vi "课堂.vi"() -> ()   [LabVIEW 2025]
panel:
  out "循环次数 3":i32
  in  "停止 2":bool
  out "x^2":dbl
  in  "数值 2":dbl
  in  "标尺.范围:最小值":dbl
  in  "标尺.范围:最大值":dbl=900.0
  in  "停止":bool
  in  "显示宽度":dbl=100.0
  in  "滑动杆":dbl(slide) scale=0.0..900.0
  out "波形图":dbl[](graph)
  in  "循环次数":i32=1000
  out "x+1 2":dbl
  out "x+1":dbl
  in  "milliseconds to wait":u32=1000
  out "数值":dbl
  out "循环次数":i32
  in  "下限":dbl=49.0
  in  "上限":dbl=51.0
  out "x/y":dbl
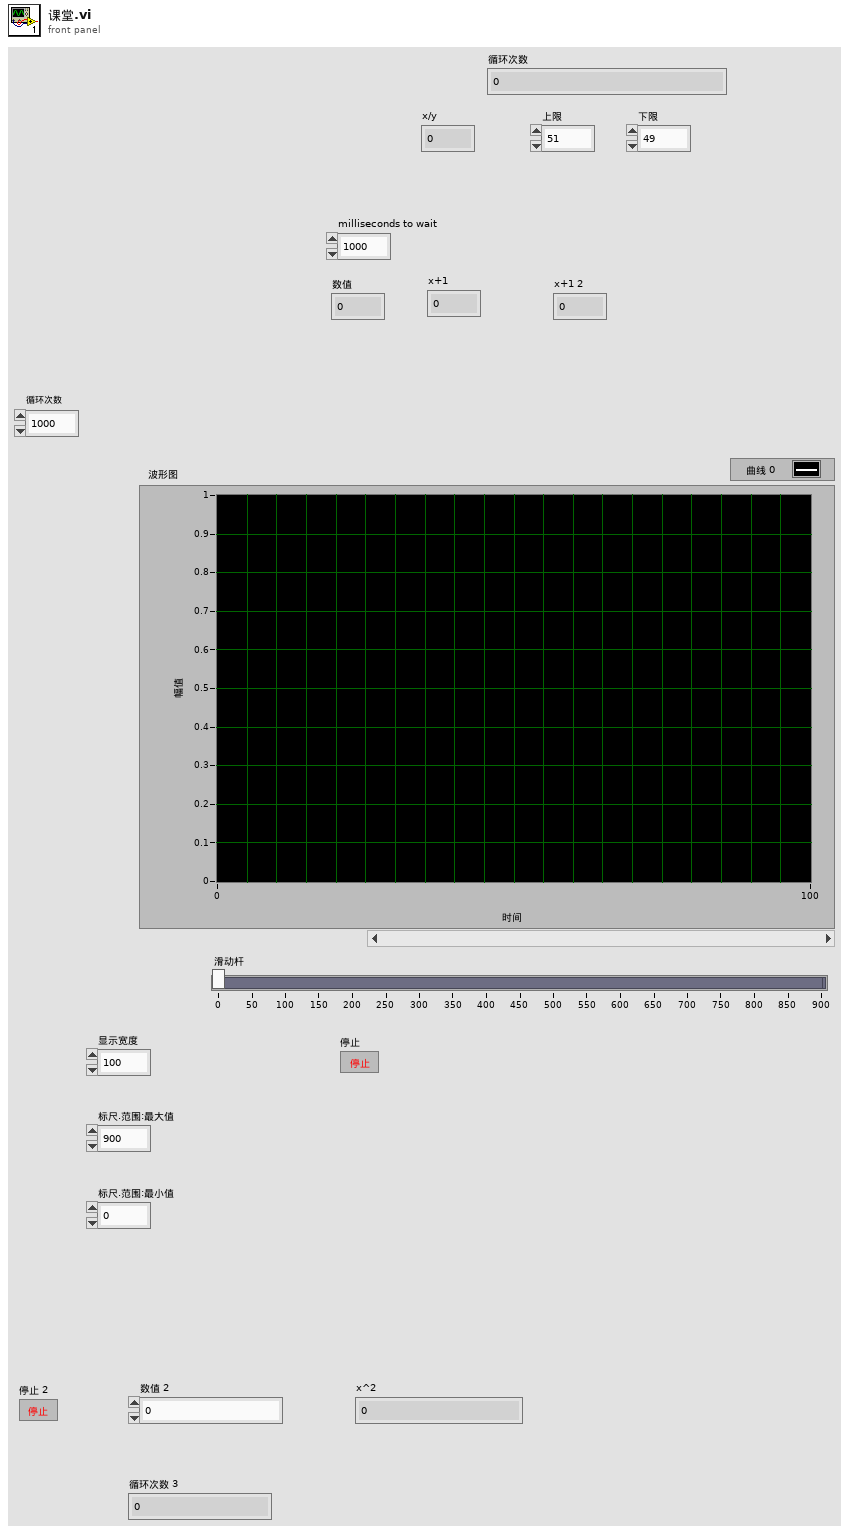
[diagram p1: front panel]
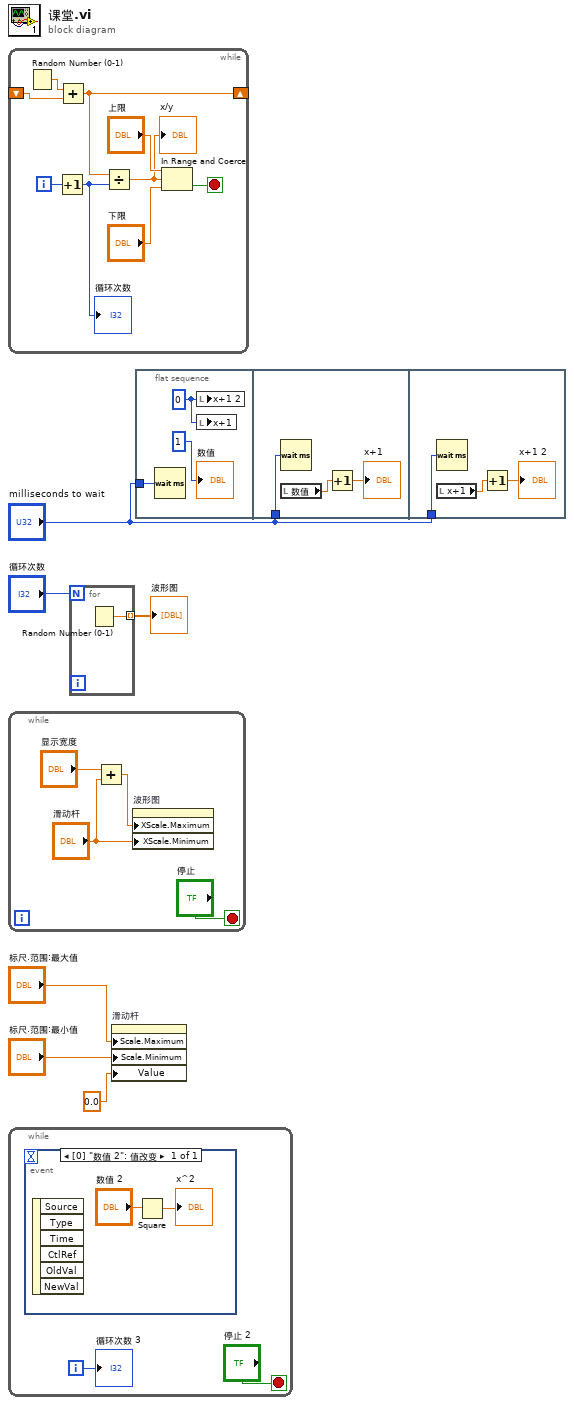
[diagram p0: block diagram]
diagram:
  n1 = while {
    shift-right: [w13] -> _
    shift-left: _ -> [w14]
    i -> [w12]
    stop <- w7 stop-if-true
    n2 = Random Number (0-1)() -> (number: 0 to 1=w15:dbl)
    n3 = Increment(x=w12) -> (x+1=w9:i32)
    "循环次数" <- w9
    n4 = Add(x=w15, y=w14) -> (x+y=w13:dbl)
    n5 = Divide(x=w13, y=w9) -> (x/y=w8:dbl)
    "x/y" <- w8
    n6 = In Range and Coerce(upper limit="上限", x=w8, lower limit="下限") -> (In Range?=w7:bool)  [unwired: 1 out]
  }
  n7 = while {
    stop <- "停止" stop-if-true
    n8 = Add(x="显示宽度", y="滑动杆") -> (x+y=w18:dbl)
    n9 = property on="波形图" class="WFGraph (严格)"("XScale.Maximum"=w18, "XScale.Minimum"="滑动杆") -> ()  [unwired: 2 in, 2 out]
  }
  n10 = while {
    i -> [w20]
    stop <- "停止 2" stop-if-true
    n11 = event shown="[0] \"数值 2\": 值改变" {
      selector: _ -> [_]
      dyn-events: _ -> [_]
      timeout: _ -> [_]
      event "数值 2": Value Change {
        n12 = event-data() -> ()  [unwired: 1 in, 6 out]
        n13 = Square(x="数值 2") -> (x^2=→"x^2":dbl)
      }
    }
    "循环次数 3" <- w20
  }
  n14 = for {
    N: "循环次数" -> [_]
    tunnel: [w24] -> w4 mode=indexing
    n15 = Random Number (0-1)() -> (number: 0 to 1=w24:dbl)
  }
  "波形图" <- w4
  n16 = property on="滑动杆" class="Slide (严格)"("Scale.Maximum"="标尺.范围:最大值", "Scale.Minimum"="标尺.范围:最小值", "Value"=0.0 ("滑动杆 2")) -> ()  [unwired: 2 in, 2 out]
  n17 = flat-sequence {
    tunnel: "milliseconds to wait" -> [w26]
    tunnel: "milliseconds to wait" -> [w30]
    tunnel: "milliseconds to wait" -> [w33]
    frame #0 {
      w25 = 0
      n18 = Wait (ms)(milliseconds to wait=w26) -> ()  [unwired: 1 out]
      n19 = local write "x+1 2"(w25) -> ()
      n20 = local write "x+1"(w25) -> ()
      "数值" <- 1
    }
    frame #1 {
      n21 = Wait (ms)(milliseconds to wait=w30) -> ()  [unwired: 1 out]
      n22 = local read "数值"() -> (w29:dbl)
      n23 = Increment(x=w29) -> (x+1=→"x+1":dbl)
    }
    frame #2 {
      n24 = Wait (ms)(milliseconds to wait=w33) -> ()  [unwired: 1 out]
      n25 = local read "x+1"() -> (w32:dbl)
      n26 = Increment(x=w32) -> (x+1=→"x+1 2":dbl)
    }
  }
